vi "Multi square wave generator.vi"() -> ()   [LabVIEW 2016]
panel:
  in  "Load array":bool
  in  "Cancel Button":bool
  out "Array":string[](array[string])
  in  "Frequency":dbl=100.0 min=100.0 max=50000.0 step=1.0 format="%#_g Hz"
  in  "GO":bool
  in  "Amplitude data":T1 {"Channel 31" min=0.0 max=102.4 step=0.012500000186264515 format="%#_g V"; "Channel 30" min=0.0 max=102.4 step=0.012500000186264515 format="%#_g V"; "Channel 29" min=0.0 max=102.4 step=0.012500000186264515 format="%#_g V"; "Channel 28" min=0.0 max=102.4 step=0.012500000186264515 format="%#_g V"; "Channel 27" min=0.0 max=102.4 step=0.012500000186264515 format="%#_g V"; "Channel 26" min=0.0 max=102.4 step=0.012500000186264515 format="%#_g V"; "Channel 25" min=0.0 max=102.4 step=0.012500000186264515 format="%#_g V"; "Channel 24" min=0.0 max=102.4 step=0.012500000186264515 format="%#_g V"; "Channel 23" min=0.0 max=102.4 step=0.012500000186264515 format="%#_g V"; "Channel 22" min=0.0 max=102.4 step=0.012500000186264515 format="%#_g V"; "Channel 21" min=0.0 max=102.4 step=0.012500000186264515 format="%#_g V"; "Channel 20" min=0.0 max=102.4 step=0.012500000186264515 format="%#_g V"; "Channel 19" min=0.0 max=102.4 step=0.012500000186264515 format="%#_g V"; "Channel 18" min=0.0 max=102.4 step=0.012500000186264515 format="%#_g V"; "Channel 17" min=0.0 max=102.4 step=0.012500000186264515 format="%#_g V"; "Channel 16" min=0.0 max=102.4 step=0.012500000186264515 format="%#_g V"; "Channel 15" min=0.0 max=102.4 step=0.012500000186264515 format="%#_g V"; "Channel 14" min=0.0 max=102.4 step=0.012500000186264515 format="%#_g V"; "Channel 13" min=0.0 max=102.4 step=0.012500000186264515 format="%#_g V"; "Channel 12" min=0.0 max=102.4 step=0.012500000186264515 format="%#_g V"; "Channel 11" min=0.0 max=102.4 step=0.012500000186264515 format="%#_g V"; "Channel 10" min=0.0 max=102.4 step=0.012500000186264515 format="%#_g V"; "Channel 9" min=0.0 max=102.4 step=0.012500000186264515 format="%#_g V"; "Channel 8" min=0.0 max=102.4 step=0.012500000186264515 format="%#_g V"; "Channel 7" min=0.0 max=102.4 step=0.012500000186264515 format="%#_g V"; "Channel 6" min=0.0 max=102.4 step=0.012500000186264515 format="%#_g V"; "Channel 5" min=0.0 max=102.4 step=0.012500000186264515 format="%#_g V"; "Channel 4" min=0.0 max=102.4 step=0.012500000186264515 format="%#_g V"; "Channel 3" min=0.0 max=102.4 step=0.012500000186264515 format="%#_g V"; "Channel 2" min=0.0 max=102.4 step=0.012500000186264515 format="%#_g V"; "Channel 1" min=0.0 max=102.4 step=0.012500000186264515 format="%#_g V"}
  in  "Arduino COM port":refnum<visa-resource-name>
  out "Status":bool
  in  "Connect":bool
  # "READ BEFORE USE"
  # "Channel 0 of AD5535 is used as voltage reference to allow the generation of biphasic squared waves (±V). \n\nDuring operation Channel 0 output is fixed at 102.4V (Vdd/2). Handle this channel correctly."
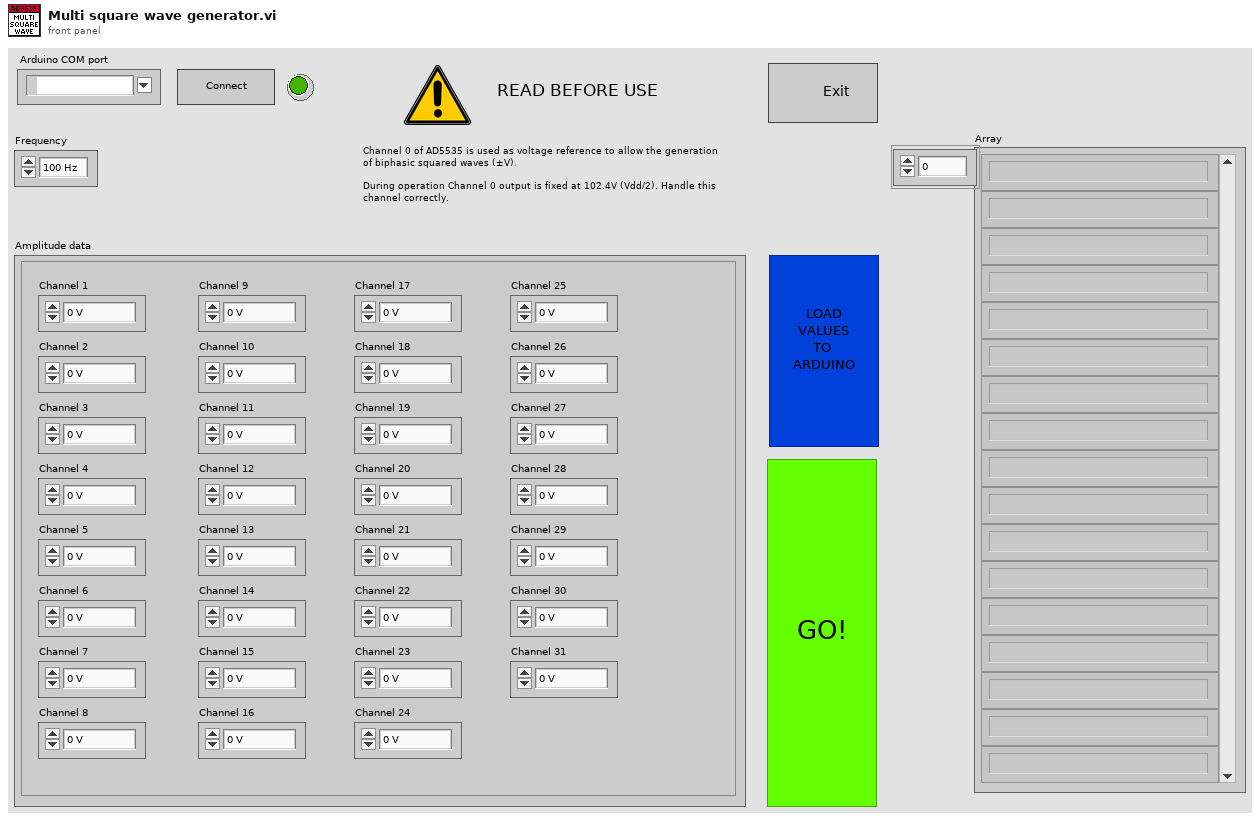
[diagram p1: front panel]
types:
  T1 = cluster{"Channel 1":dbl, "Channel 2":dbl, "Channel 3":dbl, "Channel 4":dbl, "Channel 5":dbl, "Channel 6":dbl, "Channel 7":dbl, "Channel 8":dbl, "Channel 9":dbl, "Channel 10":dbl, "Channel 11":dbl, "Channel 12":dbl, "Channel 13":dbl, "Channel 14":dbl, "Channel 15":dbl, "Channel 16":dbl, "Channel 17":dbl, "Channel 18":dbl, "Channel 19":dbl, "Channel 20":dbl, "Channel 21":dbl, "Channel 22":dbl, "Channel 23":dbl, "Channel 24":dbl, "Channel 25":dbl, "Channel 26":dbl, "Channel 27":dbl, "Channel 28":dbl, "Channel 29":dbl, "Channel 30":dbl, "Channel 31":dbl}
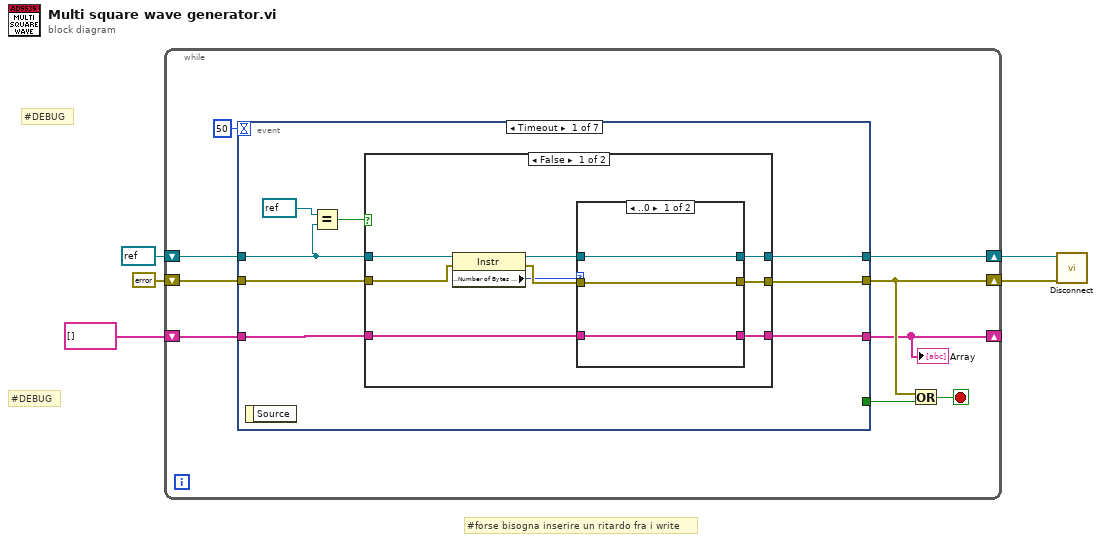
[diagram p0: block diagram]
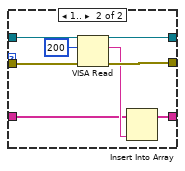
[diagram p2: hidden frame]
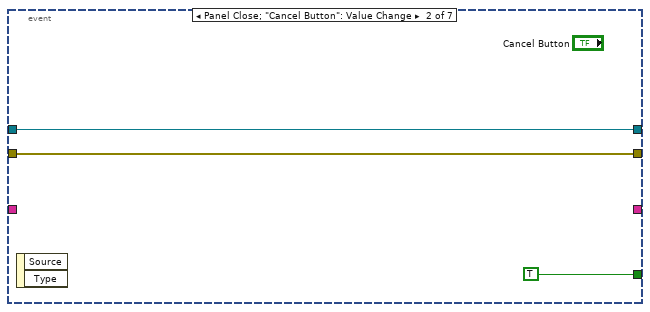
[diagram p4: hidden frame]
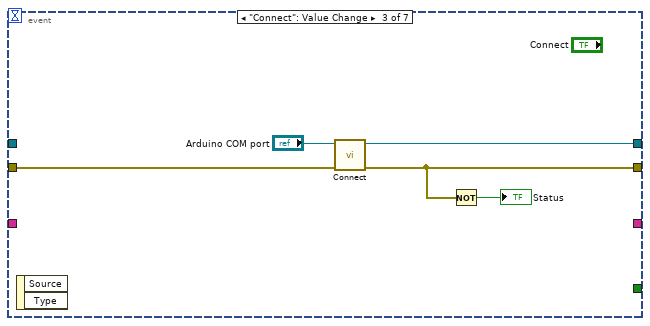
[diagram p5: hidden frame]
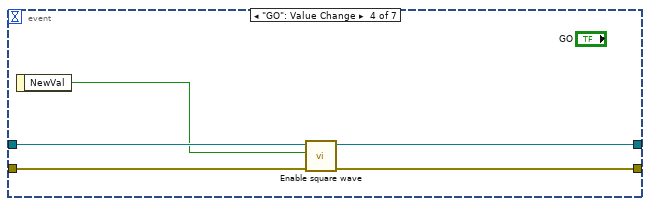
[diagram p6: hidden frame]
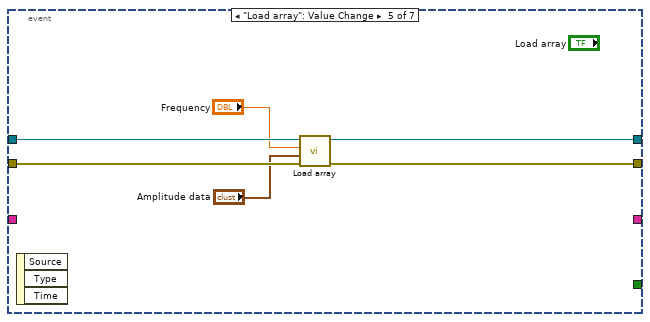
[diagram p7: hidden frame]
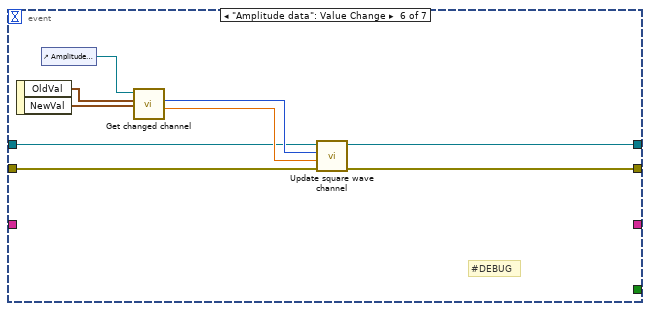
[diagram p8: hidden frame]
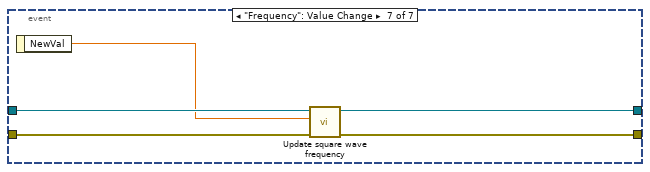
[diagram p9: hidden frame]
diagram:
  # "#DEBUG"
  # "#DEBUG"
  # "#forse bisogna inserire un ritardo fra i write"
  n1 = while {
    shift-right: [w11] -> w3
    shift-left: refnum<visa-resource-name> refnum ("Arduino Port out") -> [w10]
    shift-right: [w8] -> w2
    shift-left: errorcluster {"status"=FALSE, "code"=0, "source"=""} ("Error Out") -> [w9]
    shift-right: [w6] -> _
    shift-left: string[] [] -> [w7]
    stop <- w13 stop-if-true
    n2 = event shown="[0] Timeout" {
      selector: _ -> [_ _ _ _ _ _ _]
      dyn-events: _ -> [_ _ _ _ _ _ _]
      timeout: 50 -> [_ _ _ _ _ _ _]
      tunnel: [_ TRUE _ _ _ _ _] -> w12
      tunnel: [w20 w47 w53 w58 w62 w66 w75] -> w11
      tunnel: [w21 w46 w50 w57 w61 w65 w76] -> w8
      tunnel: w10 -> [w18 w47 _ w56 w64 w68 w78]
      tunnel: w9 -> [w22 w46 w51 w55 w63 w67 w77]
      tunnel: w7 -> [w16 _ _ _ _ _ _]
      tunnel: [w15 _ _ _ _ _ _] -> w6
      event Timeout {
        n3 = event-data() -> ()  [unwired: 1 in, 1 out]
        n4 = Equal?(x=refnum<visa-resource-name> refnum ("Arduino Port out"), y=w18) -> (x = y?=w17:bool)
        n5 = case shown="False" w17 {
          tunnel: w18 -> [w31 w45]
          tunnel: w22 -> [w28 w44]
          tunnel: [w27 w44] -> w21
          tunnel: [w26 w45] -> w20
          tunnel: w16 -> [w25 w43]
          tunnel: [w24 w43] -> w15
          frame False {
            n6 = property class="Instr"(reference=w31, error in=w28) -> (reference out=w30:refnum<visa-resource-name>, error out=w29:errorcluster, "Serial Settings:Number of Bytes at Serial Port"=w23:u32)
            n7 = case shown="..0" w23 {
              tunnel: w30 -> [w34 w42]
              tunnel: w29 -> [w33 w41]
              tunnel: [w33 w40] -> w27
              tunnel: [w34 w39] -> w26
              tunnel: w25 -> [w32 w37]
              tunnel: [w32 w36] -> w24
              frame ..0 {
              }
              frame 1.. {
                n8 = VISA Read(VISA resource name=w42, byte count=u32 200, error in (no error)=w41) -> (VISA resource name out=w39:refnum<visa-resource-name>, read buffer=w38:string, error out=w40:errorcluster)  [unwired: 1 out]
                n9 = Insert Into Array(array=w37, new element=w38) -> (w36:string[])  [unwired: 1 in]
              }
            }
          }
          frame True {
          }
        }
      }
      event Panel Close; "Cancel Button": Value Change {
        n10 = event-data() -> ()  [unwired: 1 in, 2 out]
      }
      event "Connect": Value Change {
        n11 = event-data() -> ()  [unwired: 1 in, 2 out]
        n12 = call "Connect.vi"("Error In"=w51, "Arduino Port"="Arduino COM port") -> ("Error Out"=w50:errorcluster, "Arduino Port out"=w53:refnum<visa-resource-name>)  [unwired: 8 in]
        n13 = Not(x=w50) -> (.not. x?=→"Status":bool)
      }
      event "GO": Value Change {
        n14 = event-data() -> ("NewVal"=w54:bool)  [unwired: 1 in]
        n15 = call "Enable square wave.vi"("Error In"=w55, "Enable wave"=w54, "Arduino port in"=w56) -> ("Error Out"=w57:errorcluster, "Arduino port out"=w58:refnum<visa-resource-name>)  [unwired: 7 in]
      }
      event "Load array": Value Change {
        n16 = event-data() -> ()  [unwired: 1 in, 3 out]
        n17 = call "Load array.vi"("Error In"=w63, "Amplitude data"="Amplitude data", "Frequency"="Frequency", "Arduino port in"=w64) -> ("Error Out"=w61:errorcluster, "Arduino port out"=w62:refnum<visa-resource-name>)  [unwired: 6 in]
      }
      event "Amplitude data": Value Change {
        # "#DEBUG"
        n18 = event-data() -> ("OldVal"=w72:T1, "NewVal"=w71:T1)  [unwired: 1 in]
        n19 = control-ref of="Amplitude data"() -> (w73:refnum<vi>)
        n20 = call "Get changed channel.vi"("NewVal"=w71, "OldVal"=w72, "Cluster reference"=w73) -> ("Changed value"=w69:dbl, "Changed channel"=w70:u8)  [unwired: 7 in]
        n21 = call "Update square wave channel.vi"("Error In"=w67, "Value"=w69, "Channel"=w70, "Arduino Port"=w68) -> ("Error Out"=w65:errorcluster, "Arduino Port out"=w66:refnum<visa-resource-name>)  [unwired: 6 in]
      }
      event "Frequency": Value Change {
        n22 = event-data() -> ("NewVal"=w74:dbl)  [unwired: 1 in]
        n23 = call "Update square wave frequency.vi"("Error In"=w77, "Frequency"=w74, "Arduino Port"=w78) -> ("Error Out"=w76:errorcluster, "Arduino Port out"=w75:refnum<visa-resource-name>)  [unwired: 7 in]
      }
    }
    "Array" <- w6
    n24 = Or(x=w8, y=w12) -> (x .or. y?=w13:bool)
  }
  n25 = call "Disconnect.vi"("Error In"=w2, "Arduino Port"=w3) -> ()  [unwired: 9 in, 1 out]
